vi "Get Buffer Elements.vi"(0 "Session Handle in":T1, 11 "error in (no error)":errorcluster) -> (2 "Counter":u16, 4 "Session Handle out":T1, 6 "Values":dbl[](array[numeric]), 15 "error out":errorcluster)   [LabVIEW 2015, in "Circular Buffer.lvclass"]
uses:
  Circular Buffer.lvclass
  Typedefs/Session Handle.ctl
  Circular Buffer.lvclass/Circular Buffer.ctl
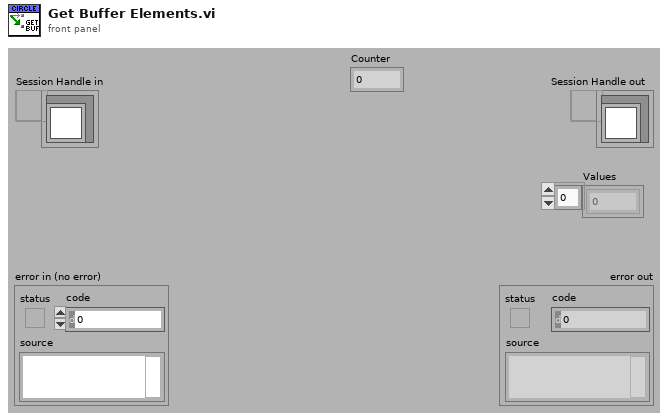
[diagram p1: front panel]
types:
  T1 = typedef "Circular Buffer.lvclass/Session Handle.ctl" = refnum<data-value>
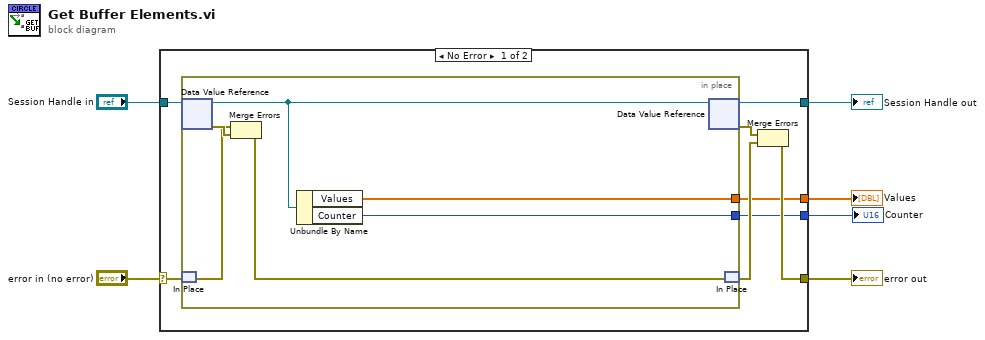
[diagram p0: block diagram]
diagram:
  n1 = case shown="No Error" "error in (no error)" {
    selector: "error in (no error)" -> [w9 w21]
    tunnel: "Session Handle in" -> [w14 w22]
    tunnel: [w13 w22] -> w5
    tunnel: [w10 w21] -> w4
    tunnel: [w8 _] -> w2
    tunnel: [w7 _] -> w1
    frame No Error {
      n2 = in-place {
        in-place-border: [w16] -> w8
        in-place-border: [w15] -> w7
        n3 = in-place-dvr #1(w14) -> (w17:refnum<class "Circular Buffer.lvclass">, w19:errorcluster)
        n4 = in-place-match #2(w9) -> (w18:errorcluster)
        n5 = Merge Errors(w18, w19) -> (w20:errorcluster)
        n6 = Unbundle By Name(w17) -> ("Values"=w16:dbl[], "Counter"=w15:u16)
        n7 = in-place-dvr #1(w17) -> (w13:T1, w11:errorcluster)
        n8 = in-place-match #2(w20) -> (w12:errorcluster)
      }
      n9 = Merge Errors(w11, w12) -> (w10:errorcluster)
    }
    frame Error {
    }
  }
  "Session Handle out" <- w5
  "error out" <- w4
  "Values" <- w2
  "Counter" <- w1
